vi "重置信息.vi"(0 "MainPage 输入":refnum<class "MainPage.lvclass">, 10 "连接方式":enum16{"网口(客服端)", "网口(服务端)", "串口"}(ring)) -> (14 "MainPage 输出":refnum<class "MainPage.lvclass">)   [LabVIEW 2019, in "MainPage.lvlib" / "MainPage.lvclass"]
uses:
  MainPage.lvclass
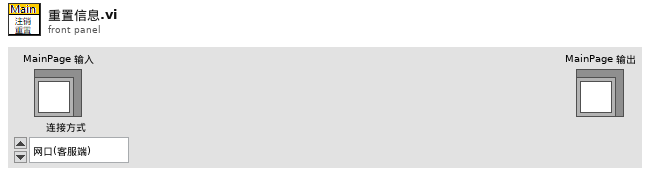
[diagram p1: front panel]
types:
  T1 = typedef "MainPage.lvlib/MainPage.lvclass/DataRef_通讯接口.ctl" = cluster{"连接方式":enum16{"网口(客服端)", "网口(服务端)", "串口"}, "VISA串口名称":refnum<visa-resource-name>, "服务端识别":cluster{"本机IP":string, "本机端口":u16, "当前目标":string}, "客服端识别":cluster{"客P-主IP:Port":string}, "服务端记录":cluster{"服务端侦听ID":refnum<k5>, "服务端接口记录":map{string, refnum<k5>}}, "客服端记录":map{string, refnum<k5>}}
  T2 = enum16{"ini", "读取", "写入-报文记录", "写入-寄存器模拟", "写入-串口状态", "增加报文记录"}
  T3 = enum16{"ini", "增加记录", "读取记录", "更改寄存器值", "更改接口状态", "更改报文信息", "增加报文信息"}
  T4 = typedef "MainPage.lvlib/MainPage.lvclass/通用配置选项.ctl" = cluster{"ModBusRTU反馈":enum32{"模拟反馈", "无反馈", "错误反馈"}, "侦听周期":u32, "跳转反馈":bool, "报文记录数量":u16, "客服端新增模式":enum32{"单端模式", "多端共存"}}
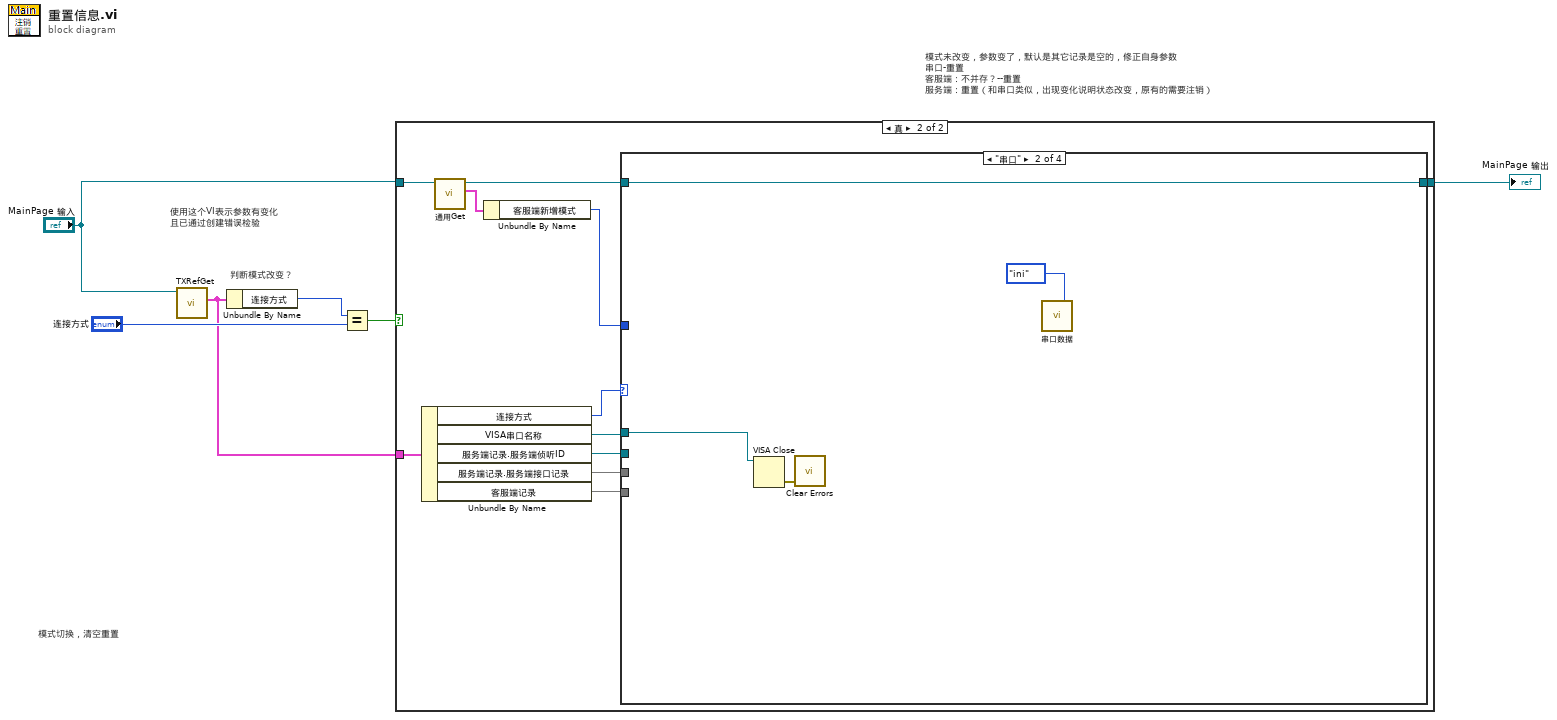
[diagram p0: block diagram]
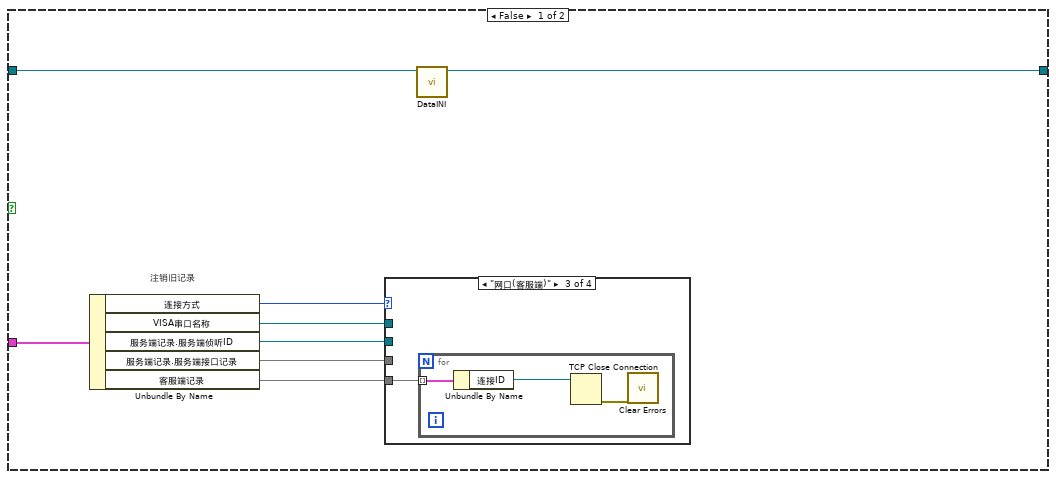
[diagram p2: hidden frame]
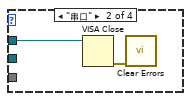
[diagram p4: hidden frame]
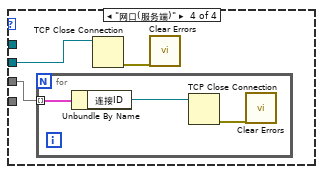
[diagram p5: hidden frame]
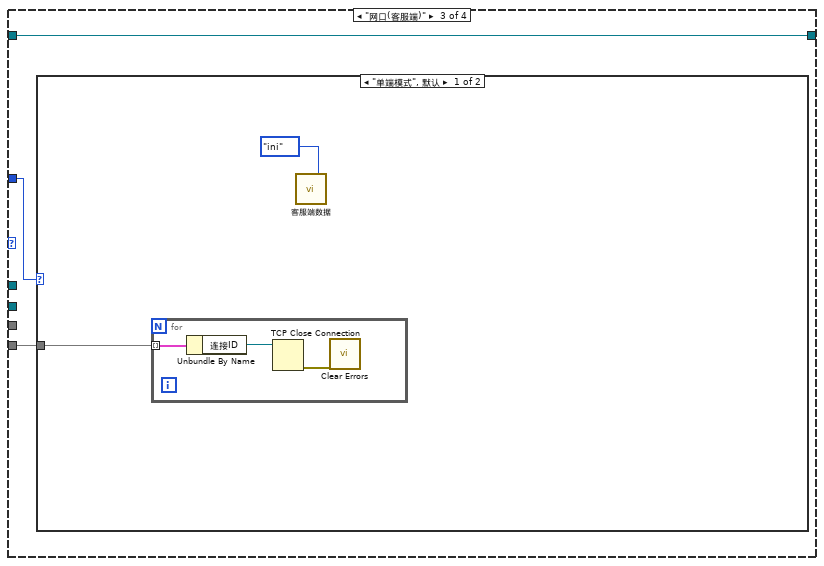
[diagram p7: hidden frame]
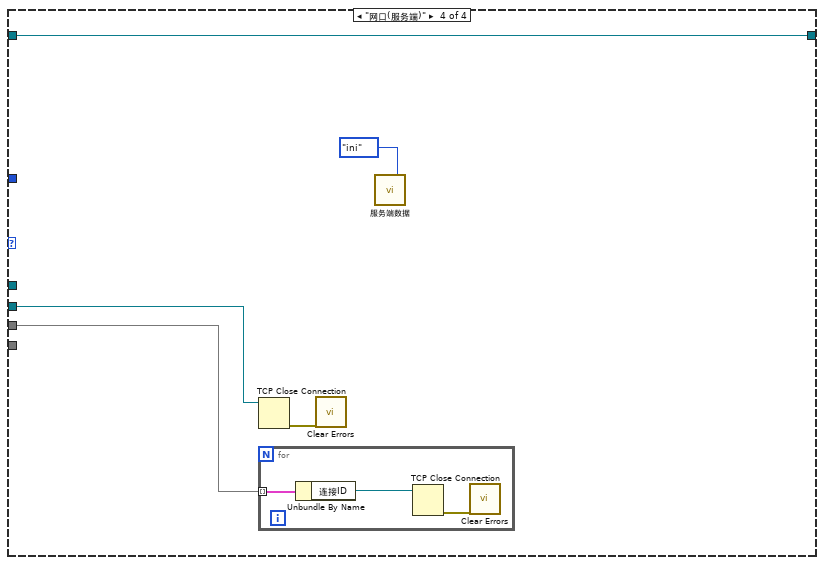
[diagram p9: hidden frame]
diagram:
  # "模式未改变，参数变了，默认是其它记录是空的，修正自身参数\n串口-重置\n客服端：不并存？--重置\n服务端：重置（和串口类似，出现变化说明状态改变，原有的需要注销）"
  # "模式切换，清空重置"
  # "使用这个VI表示参数有变化\n且已通过创建错误检验"
  # "判断模式改变？"
  n1 = call-dynamic "TXRefGet.vi"("MainPage 输入"="MainPage 输入") -> ("通讯接口数据"=w2:T1)  [unwired: 6 in, 4 out]
  n2 = Unbundle By Name(w2) -> ("连接方式"=w6:enum16{"网口(客服端)", "网口(服务端)", "串口"})
  n3 = Equal?(x=w6, y="连接方式") -> (x = y?=w5:bool)
  n4 = case shown="真" w5 {
    tunnel: "MainPage 输入" -> [w8 w31]
    tunnel: [w7 w27] -> w4
    tunnel: w2 -> [w14 w37]
    frame False {
      # "注销旧记录"
      n5 = Unbundle By Name(w14) -> ("连接方式"=w13:enum16{"网口(客服端)", "网口(服务端)", "串口"}, "VISA串口名称"=w12:refnum<visa-resource-name>, "服务端记录.服务端侦听ID"=w10:refnum<k5>, "服务端记录.服务端接口记录"=w9:map{string, refnum<k5>}, "客服端记录"=w11:map{string, refnum<k5>})
      n6 = case shown="\"网口(客服端)\"" w13 {
        tunnel: w12 -> [_ w16 _ _]
        tunnel: w11 -> [_ _ w17 _]
        tunnel: w10 -> [_ _ _ w21]
        tunnel: w9 -> [_ _ _ w23]
        frame Default {
        }
        frame "串口" {
          n7 = VISA Close(VISA resource name=w16) -> (error out=w15:errorcluster)  [unwired: 1 in]
          n8 = call <vilib>:"Clear Errors.vi"("error in (no error)"=w15) -> ()  [unwired: 5 in, 2 out]
        }
        frame "网口(客服端)" {
          n9 = for {
            tunnel: w17 -> [w20] mode=indexing
            n10 = Unbundle By Name(w20) -> ("连接ID"=w19:refnum<k5>)
            n11 = TCP Close Connection(connection ID=w19) -> (error out=w18:errorcluster)  [unwired: 2 in, 1 out]
            n12 = call <vilib>:"Clear Errors.vi"("error in (no error)"=w18) -> ()  [unwired: 5 in, 2 out]
          }
        }
        frame "网口(服务端)" {
          n13 = for {
            tunnel: w23 -> [w26] mode=indexing
            n14 = Unbundle By Name(w26) -> ("连接ID"=w25:refnum<k5>)
            n15 = TCP Close Connection(connection ID=w25) -> (error out=w24:errorcluster)  [unwired: 2 in, 1 out]
            n16 = call <vilib>:"Clear Errors.vi"("error in (no error)"=w24) -> ()  [unwired: 5 in, 2 out]
          }
          n17 = TCP Close Connection(connection ID=w21) -> (error out=w22:errorcluster)  [unwired: 2 in, 1 out]
          n18 = call <vilib>:"Clear Errors.vi"("error in (no error)"=w22) -> ()  [unwired: 5 in, 2 out]
        }
      }
      n19 = call-dynamic "DataINI.vi"("MainPage 输入"=w8) -> ("MainPage 输出"=w7:refnum<class "MainPage.lvclass">)  [unwired: 9 in, 1 out]
    }
    frame True {
      n20 = Unbundle By Name(w37) -> ("连接方式"=w36:enum16{"网口(客服端)", "网口(服务端)", "串口"}, "VISA串口名称"=w35:refnum<visa-resource-name>, "服务端记录.服务端侦听ID"=w34:refnum<k5>, "服务端记录.服务端接口记录"=w33:map{string, refnum<k5>}, "客服端记录"=w32:map{string, refnum<k5>})
      n21 = call-dynamic "通用Get.vi"("MainPage 输入"=w31) -> ("通用配置"=w30:T4, "MainPage 输出"=w28:refnum<class "MainPage.lvclass">)  [unwired: 6 in, 3 out]
      n22 = Unbundle By Name(w30) -> ("客服端新增模式"=w29:enum32{"单端模式", "多端共存"})
      n23 = case shown="\"串口\"" w36 {
        tunnel: w35 -> [_ w41 _ _]
        tunnel: w32 -> [_ _ w43 _]
        tunnel: w34 -> [_ _ _ w53]
        tunnel: w33 -> [_ _ _ w55]
        tunnel: w29 -> [_ _ w45 _]
        tunnel: w28 -> [w38 w40 w44 w52]
        tunnel: [w38 w40 w44 w52] -> w27
        frame Default {
        }
        frame "串口" {
          n24 = VISA Close(VISA resource name=w41) -> (error out=w42:errorcluster)  [unwired: 1 in]
          n25 = call <vilib>:"Clear Errors.vi"("error in (no error)"=w42) -> ()  [unwired: 5 in, 2 out]
          n26 = call "串口数据.vi"("枚举"=T2."ini") -> ()  [unwired: 18 in, 1 out]
        }
        frame "网口(客服端)" {
          n27 = case shown="\"单端模式\", 默认" w45 {
            tunnel: w43 -> [w47 _]
            frame "单端模式", Default {
              n28 = for {
                tunnel: w47 -> [w50] mode=indexing
                n29 = Unbundle By Name(w50) -> ("连接ID"=w49:refnum<k5>)
                n30 = TCP Close Connection(connection ID=w49) -> (error out=w48:errorcluster)  [unwired: 2 in, 1 out]
                n31 = call <vilib>:"Clear Errors.vi"("error in (no error)"=w48) -> ()  [unwired: 5 in, 2 out]
              }
              n32 = call "客服端数据.vi"("枚举"=T3."ini") -> ()  [unwired: 17 in, 2 out]
            }
            frame "多端共存" {
            }
          }
        }
        frame "网口(服务端)" {
          n33 = TCP Close Connection(connection ID=w53) -> (error out=w54:errorcluster)  [unwired: 2 in, 1 out]
          n34 = for {
            tunnel: w55 -> [w58] mode=indexing
            n35 = Unbundle By Name(w58) -> ("连接ID"=w57:refnum<k5>)
            n36 = TCP Close Connection(connection ID=w57) -> (error out=w56:errorcluster)  [unwired: 2 in, 1 out]
            n37 = call <vilib>:"Clear Errors.vi"("error in (no error)"=w56) -> ()  [unwired: 5 in, 2 out]
          }
          n38 = call <vilib>:"Clear Errors.vi"("error in (no error)"=w54) -> ()  [unwired: 5 in, 2 out]
          n39 = call "服务端数据.vi"("枚举"=T3."ini") -> ()  [unwired: 17 in, 2 out]
        }
      }
    }
  }
  "MainPage 输出" <- w4
